vi "practice6.vi"() -> ()   [LabVIEW 2018]
panel:
  out "数値 2":dbl
  in  "数値":dbl
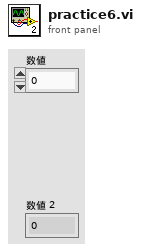
[diagram p1: front panel]
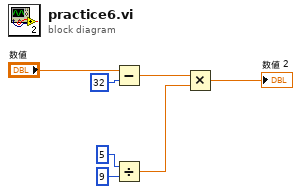
[diagram p0: block diagram]
diagram:
  n1 = Subtract(x="数値", y=32) -> (x-y=w3:dbl)
  n2 = Divide(x=5, y=9) -> (x/y=w2:dbl)
  n3 = Multiply(x=w3, y=w2) -> (x*y=→"数値 2":dbl)
